vi "Is File a LabVIEW document.vi"(8 "error in (no error)":errorcluster, 11 "path":path) -> (0 "error out":errorcluster, 3 "Is LabVIEW document?":bool)   [LabVIEW 2014, in "NI_FileType.lvlib"]
doc: "Returns TRUE if this file could be opened by LabVIEW. It uses the same criteria as the File >> Open dialog."
uses:
  NI_FileType.lvlib
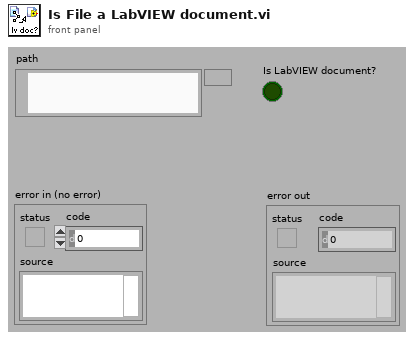
[diagram p1: front panel]
types:
  T1 = typedef "NI_FileType.lvlib/FT_FileTypes.ctl" = enum32{"Invalid file/path", "Unknown type", "Instrument", "Control", "Polymorphic VI", "Project", "Library", "LVClass", "XControl", "XNode", "CIN", "Run-time menu", "Palette menu", "LLB", "Shortcut", "Directory", "Class Private Data Control", "Statechart", "MathScript .m file", "Ladder Diagram", "LVLibp"}
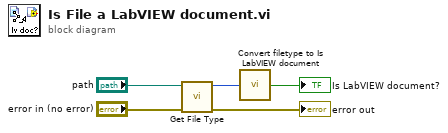
[diagram p0: block diagram]
diagram:
  n1 = call "Get File Type.vi"("error in (no error)"="error in (no error)", "path"="path") -> ("error out"=→"error out":errorcluster, "file type"=w2:T1)  [unwired: 7 in, 1 out]
  n2 = call "Convert filetype to Is LabVIEW document.vi"("file type"=w2) -> ("Is LabVIEW document?"=→"Is LabVIEW document?":bool)  [unwired: 4 in]
